vi "OperatorControlBox_XControl_Facade.vi"(0 "Data In":T4, 2 "Display State In":T2, 3 "Container State":T3) -> (6 "Data Out":T4, 7 "Display State Out":T2, 8 "Action":T1)   [LabVIEW 2018, in "OperatorControlBox_XControl.xctl"]
uses:
  OperatorControlBox_XControl.xctl
  OperatorControlBox_XControl_Data.ctl
  General/OperatorControlBox/TypeDefs/OperatorControlBoxButtons_Type.ctl
  <vilib>/_xctls/Container State.ctl
  OperatorControlBox_XControl_State.ctl
  <vilib>/_xctls/Action.ctl
  General/OperatorControlBox/TypeDefs/OperatorControlBoxButtonPosition_Type.ctl
  <vilib>/_xctls/XControlSupport.lvlib
panel:
  out "LED_Left":bool
  out "LED_Right":bool
  in  "Left_Right":bool
  out "LED_Cargo":bool
  out "LED_Hatch":bool
  in  "Hatch_Cargo":bool
  out "LED_Button4":bool
  in  "Button4":bool
  out "LED_Button3":bool
  in  "Button3":bool
  out "LED_Button2":bool
  in  "Button2":bool
  out "LED_Button1":bool
  in  "Button1":bool
  out "LED_Switch1_Right":bool
  out "LED_Switch1_Left":bool
  in  "Switch1":bool
  out "LED_Switch2_Right":bool
  out "LED_Switch2_Left":bool
  in  "Switch2":bool
  out "LED_Climb":bool
  in  "Climb":bool
  out "LED_CargoShip":bool
  in  "CargoShip":bool
  out "LED_Depot":bool
  in  "Depot":bool
  out "LED_FeederStation":bool
  in  "FeederStation":bool
  out "LED_NearRocketHigh":bool
  in  "NearRocketHigh":bool
  out "LED_NearRocketMid":bool
  in  "NearRocketMid":bool
  out "LED_NearRocketLow":bool
  in  "NearRocketLow":bool
  out "LED_FarRocketHigh":bool
  in  "FarRocketHigh":bool
  out "LED_FarRocketMid":bool
  in  "FarRocketMid":bool
  out "LED_FarRocketLow":bool
  in  "FarRocketLow":bool
  # "Left"
  # "Right"
  # "Hatch"
  # "Cargo"
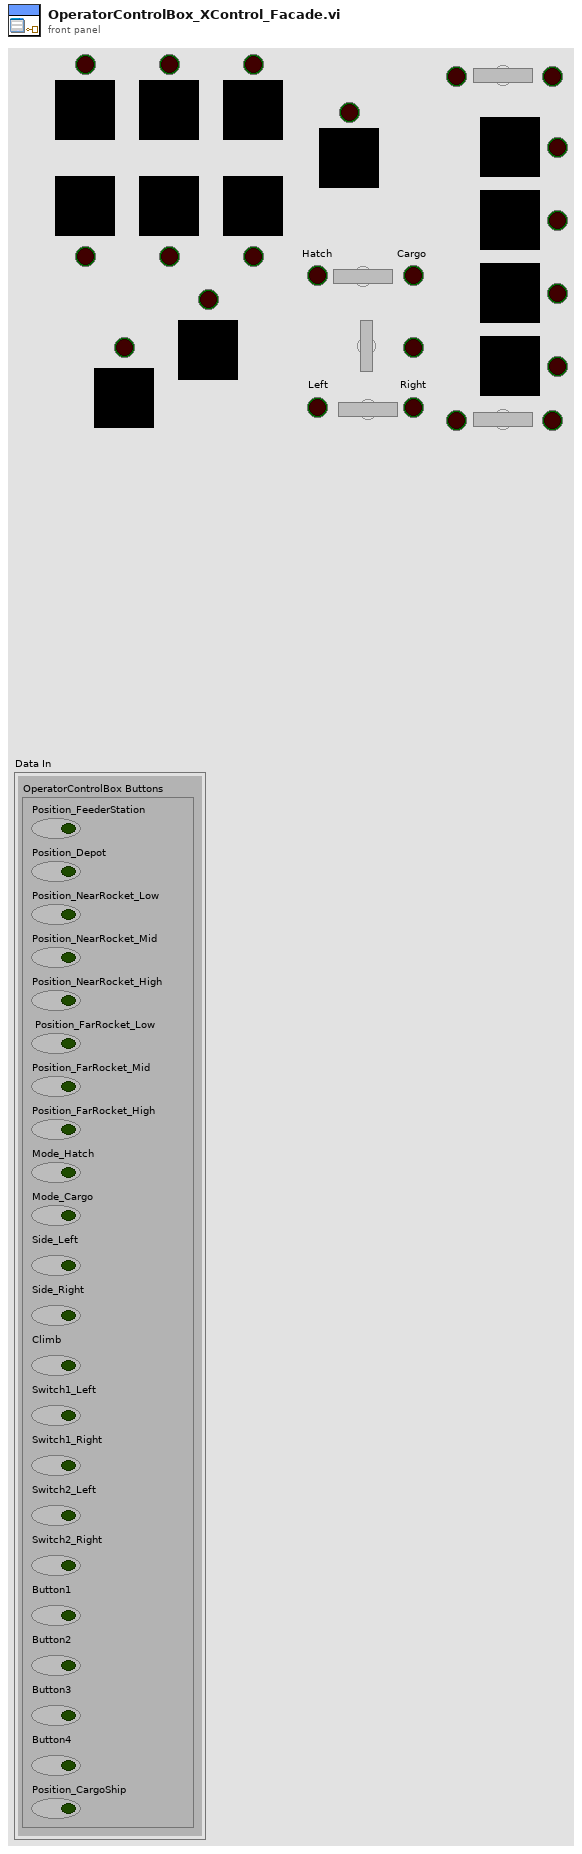
[diagram p1: front panel]
types:
  T1 = typedef "XControlSupport.lvlib/Action.ctl" = cluster{"Data Changed?":bool, "State Changed?":bool, "Action Name":string}
  T2 = typedef "OperatorControlBox_XControl.xctl/OperatorControlBox_XControl_State.ctl" = cluster{"Numeric":dbl}
  T3 = typedef "XControlSupport.lvlib/Container State.ctl" = cluster{"Indicator?":bool, "Run Mode?":bool, " Refnum":refnum<vi>}
  T4 = typedef "OperatorControlBox_XControl.xctl/OperatorControlBox_XControl_Data.ctl" = cluster{"OperatorControlBox Buttons":T5}
  T5 = typedef "OperatorControlBoxButtons_Type.ctl" = cluster{"Position_FeederStation":bool, "Position_Depot":bool, "Position_NearRocket_Low":bool, "Position_NearRocket_Mid":bool, "Position_NearRocket_High":bool, " Position_FarRocket_Low":bool, "Position_FarRocket_Mid":bool, "Position_FarRocket_High":bool, "Mode_Hatch":bool, "Mode_Cargo":bool, "Side_Left":bool, "Side_Right":bool, "Climb":bool, "Switch1_Left":bool, "Switch1_Right":bool, "Switch2_Left":bool, "Switch2_Right":bool, "Button1":bool, "Button2":bool, "Button3":bool, "Button4":bool, "Position_CargoShip":bool}
  T6 = typedef "OperatorControlBoxButtonPosition_Type.ctl" = enum16{"Unknown", "FeederStation", "Depot", "NearRocketLow", "NearRocketMid", "NearRocketHigh", "FarRocketLow", "FarRocketMid", "FarRocketHigh", "CargoShip"}
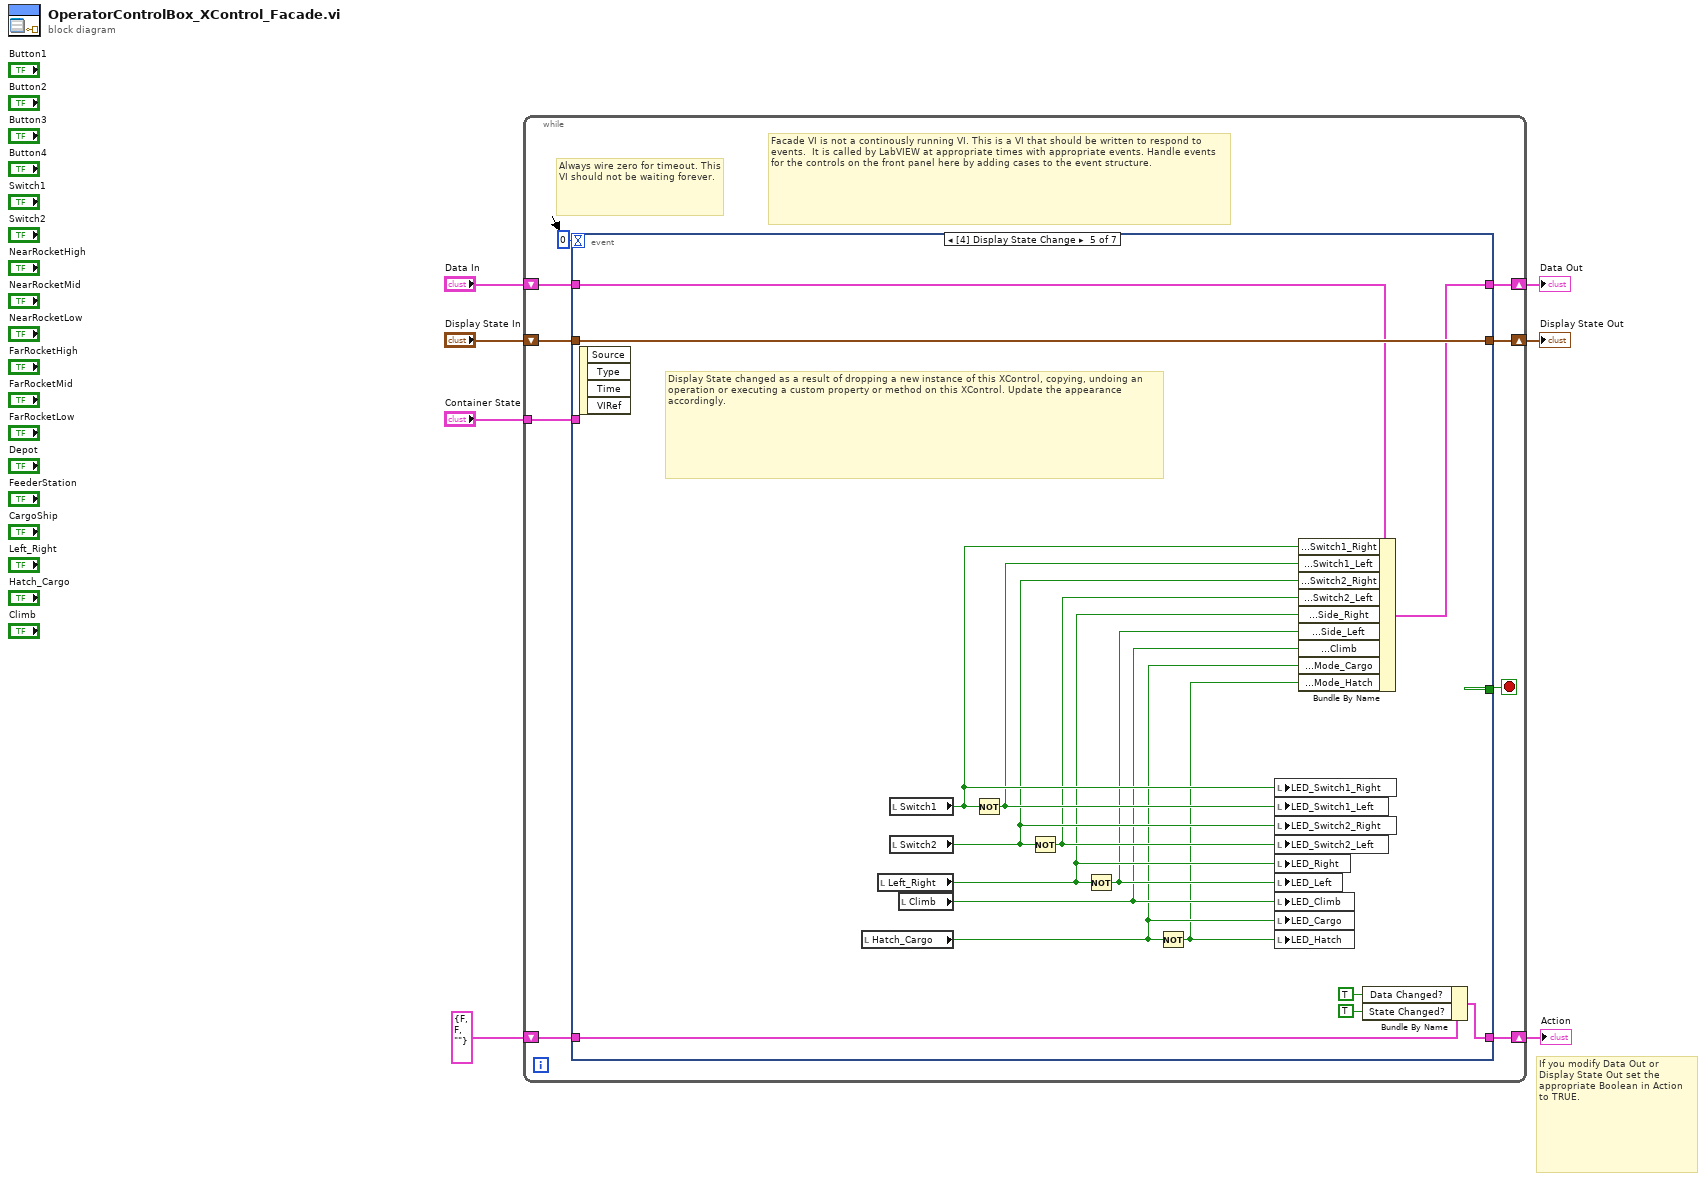
[diagram p0: block diagram]
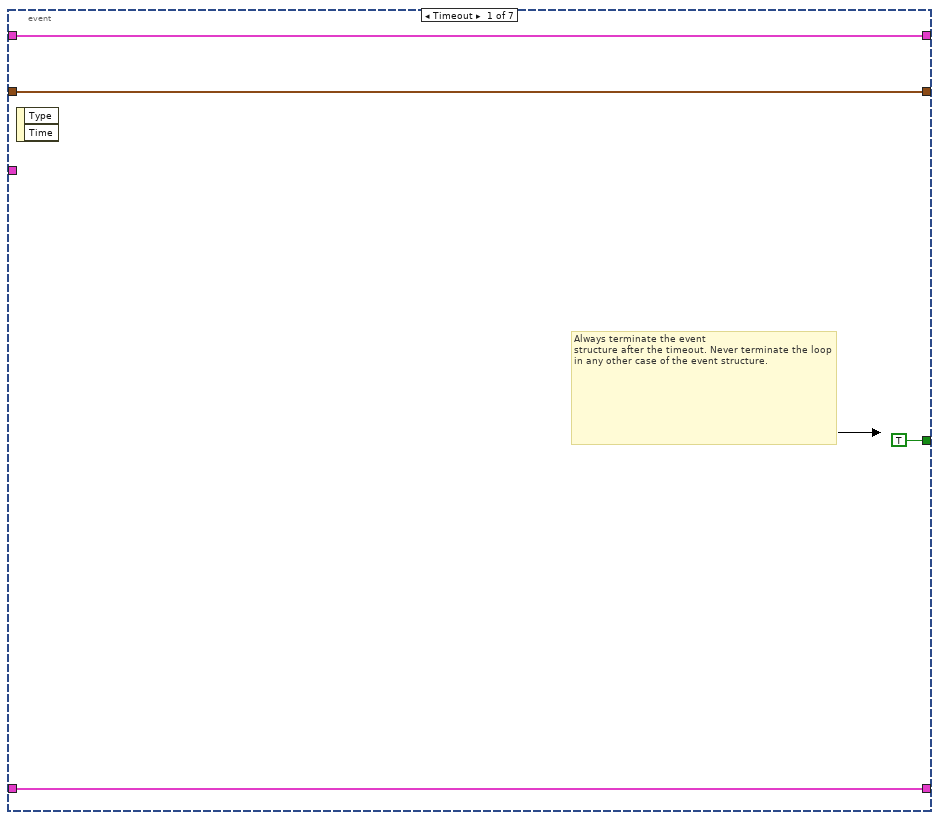
[diagram p2: hidden frame]
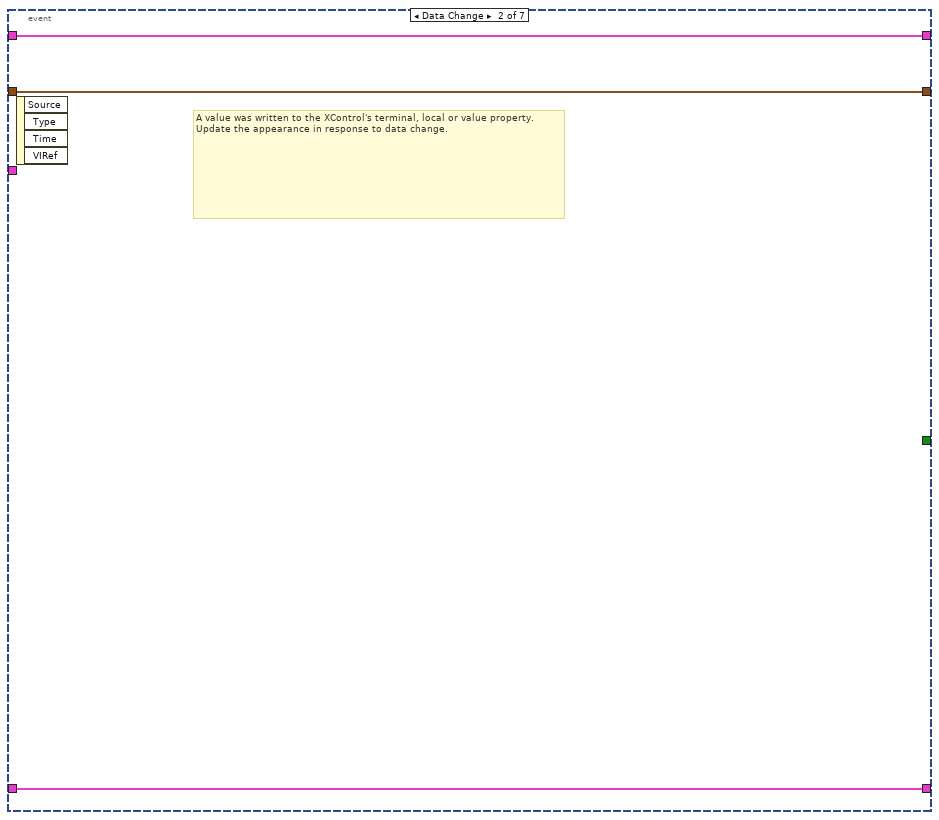
[diagram p3: hidden frame]
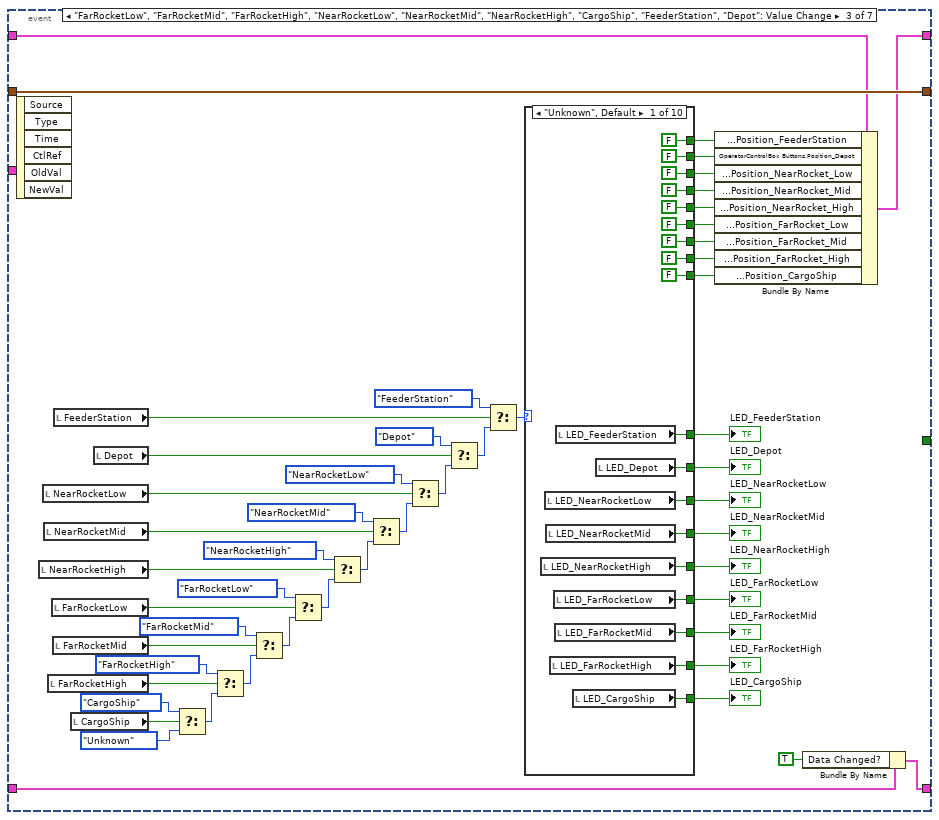
[diagram p4: hidden frame]
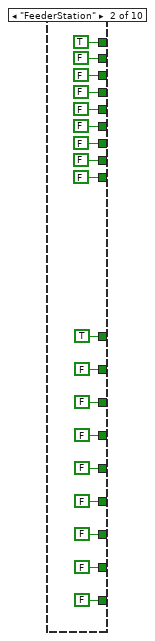
[diagram p5: hidden frame]
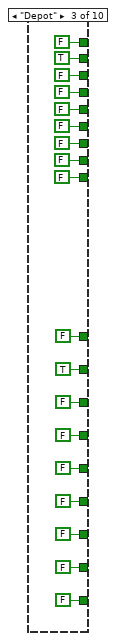
[diagram p6: hidden frame]
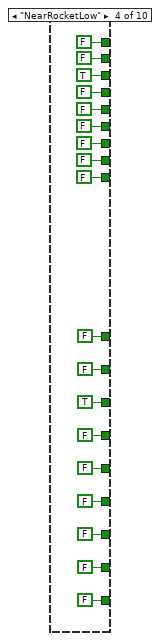
[diagram p7: hidden frame]
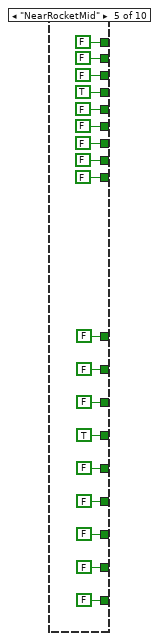
[diagram p8: hidden frame]
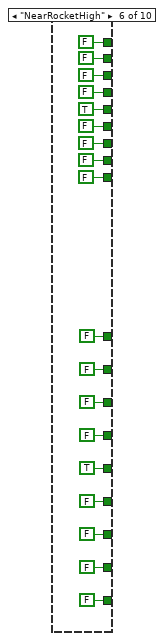
[diagram p9: hidden frame]
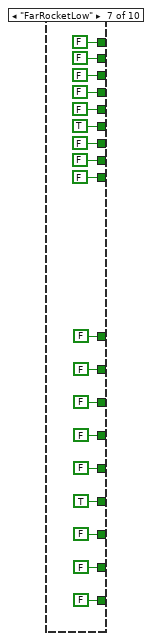
[diagram p10: hidden frame]
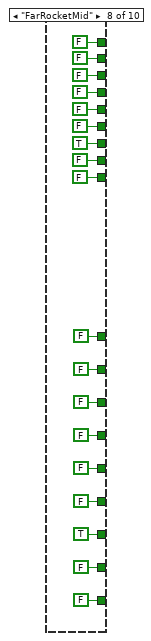
[diagram p11: hidden frame]
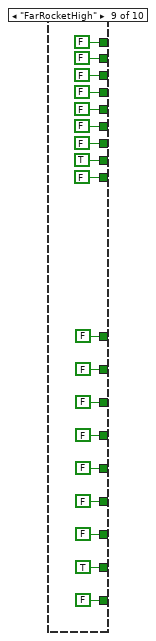
[diagram p12: hidden frame]
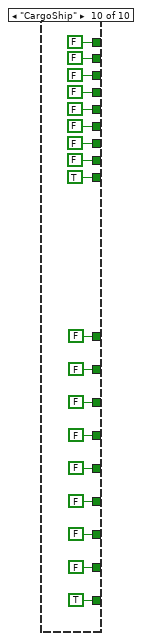
[diagram p13: hidden frame]
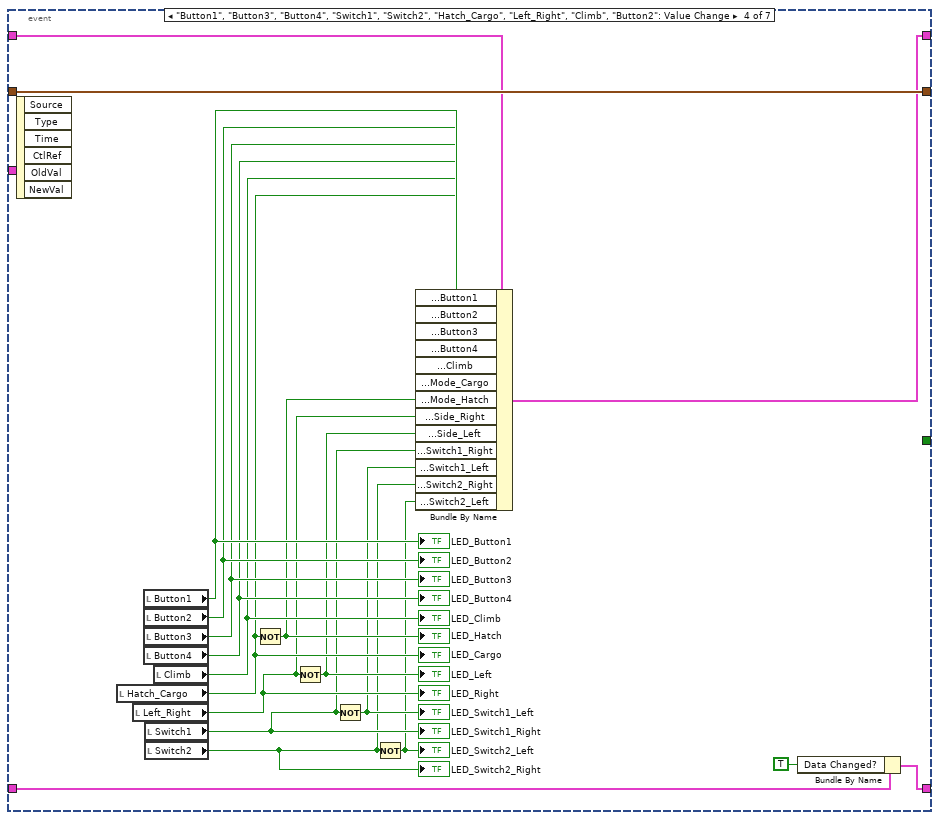
[diagram p14: hidden frame]
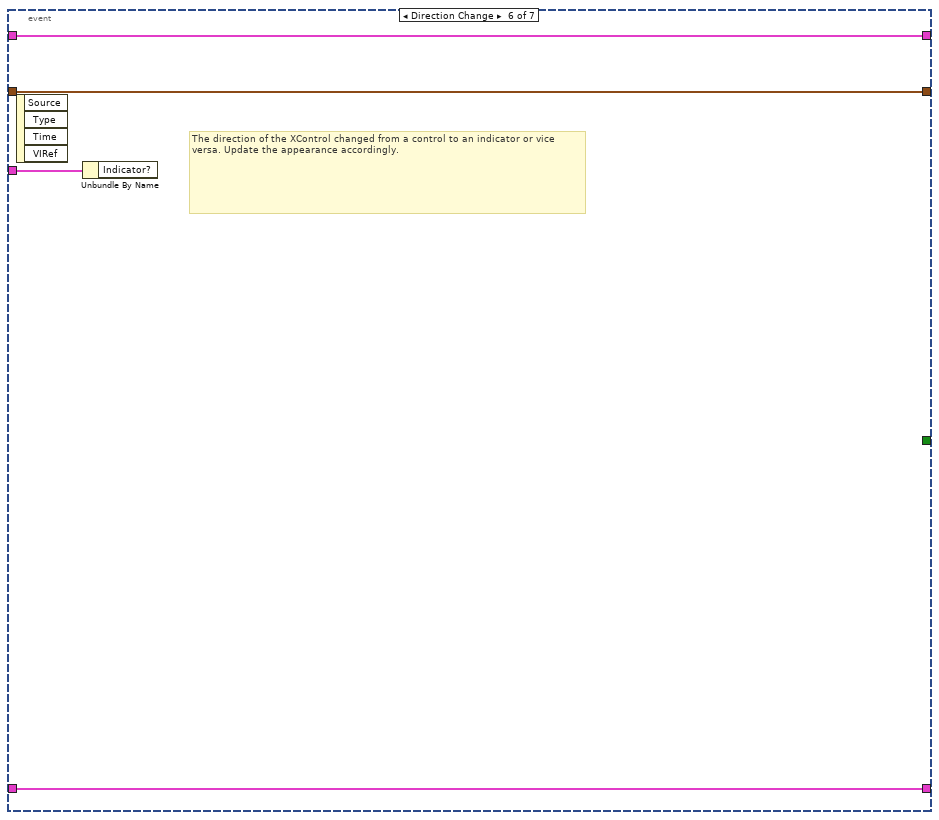
[diagram p15: hidden frame]
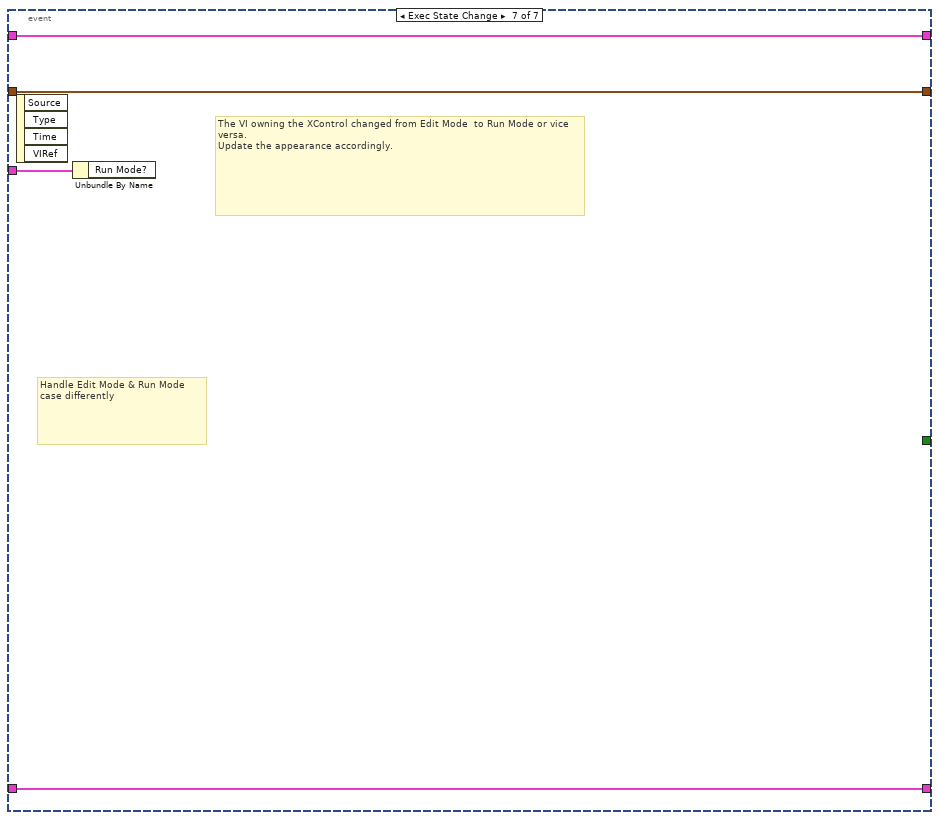
[diagram p16: hidden frame]
diagram:
  # "If you modify Data Out or\nDisplay State Out set the\nappropriate Boolean in Action\nto TRUE."
  n1 = while {
    shift-right: [w15] -> w4
    shift-left: "Display State In" -> [w16]
    tunnel: "Container State" -> [w12]
    shift-right: [w10] -> w7
    shift-left: "Data In" -> [w11]
    shift-right: [w8] -> w2
    shift-left: T1 {"Data Changed?"=FALSE, "State Changed?"=FALSE, "Action Name"=""} ("Action") -> [w9]
    stop <- w14 stop-if-true
    # "Facade VI is not a continously running VI. This is a VI that should be written to respond to events.  It is called by LabVIEW at appropriate times with appropriate events. Handle events for the controls on the front panel here by adding cases to the event structure."
    # "Always wire zero for timeout. This\nVI should not be waiting forever."
    n2 = event shown="[4] Display State Change" {
      selector: _ -> [_ _ _ _ _ _ _]
      dyn-events: _ -> [_ _ _ _ _ _ _]
      timeout: 0 -> [_ _ _ _ _ _ _]
      tunnel: w16 -> [w18 w22 w75 w274 w290 w293 w297]
      tunnel: [w18 w22 w75 w274 w290 w293 w297] -> w15
      tunnel: [TRUE _ _ _ _ _ _] -> w14
      tunnel: w12 -> [_ _ _ _ _ w294 w298]
      tunnel: w11 -> [w17 w23 w50 w273 w289 w292 w296]
      tunnel: [w17 w23 w49 w272 w288 w292 w296] -> w10
      tunnel: [w19 w21 w25 w256 w275 w291 w295] -> w8
      tunnel: w9 -> [w19 w21 w26 w257 w276 w291 w295]
      event Timeout {
        # "Always terminate the event\nstructure after the timeout. Never terminate the loop in any other case of the event structure."
        n3 = event-data() -> ()  [unwired: 1 in, 2 out]
      }
      event Data Change {
        # "A value was written to the XControl's terminal, local or value property.\nUpdate the appearance in response to data change."
        n4 = event-data() -> ()  [unwired: 1 in, 4 out]
      }
      event "FarRocketLow", "FarRocketMid", "FarRocketHigh", "NearRocketLow", "NearRocketMid", "NearRocketHigh", "CargoShip", "FeederStation", "Depot": Value Change {
        n5 = event-data() -> ()  [unwired: 1 in, 6 out]
        n6 = local read "NearRocketHigh"() -> (w56:bool)
        n7 = local read "NearRocketLow"() -> (w54:bool)
        n8 = local read "NearRocketMid"() -> (w55:bool)
        n9 = local read "FarRocketHigh"() -> (w74:bool)
        n10 = local read "FarRocketLow"() -> (w57:bool)
        n11 = local read "FarRocketMid"() -> (w58:bool)
        n12 = local read "FeederStation"() -> (w52:bool)
        n13 = local read "CargoShip"() -> (w30:bool)
        n14 = local read "Depot"() -> (w53:bool)
        n15 = Select(t=OperatorControlBoxButtonPosition_Type."CargoShip", s=w30, f=OperatorControlBoxButtonPosition_Type."Unknown") -> (s? t:f=w28:T6)
        n16 = Select(t=OperatorControlBoxButtonPosition_Type."FarRocketHigh", s=w74, f=w28) -> (s? t:f=w71:T6)
        n17 = Select(t=OperatorControlBoxButtonPosition_Type."FarRocketMid", s=w58, f=w71) -> (s? t:f=w69:T6)
        n18 = Select(t=OperatorControlBoxButtonPosition_Type."FarRocketLow", s=w57, f=w69) -> (s? t:f=w67:T6)
        n19 = Select(t=OperatorControlBoxButtonPosition_Type."NearRocketHigh", s=w56, f=w67) -> (s? t:f=w65:T6)
        n20 = Select(t=OperatorControlBoxButtonPosition_Type."NearRocketMid", s=w55, f=w65) -> (s? t:f=w63:T6)
        n21 = Select(t=OperatorControlBoxButtonPosition_Type."NearRocketLow", s=w54, f=w63) -> (s? t:f=w61:T6)
        n22 = Select(t=OperatorControlBoxButtonPosition_Type."Depot", s=w53, f=w61) -> (s? t:f=w59:T6)
        n23 = Select(t=OperatorControlBoxButtonPosition_Type."FeederStation", s=w52, f=w59) -> (s? t:f=w51:T6)
        n24 = case shown="\"Unknown\", Default" w51 {
          tunnel: [FALSE ("OperatorControlBox Buttons.Position_FeederStation") TRUE ("OperatorControlBox Buttons.Position_FeederStation") FALSE ("OperatorControlBox Buttons.Position_FeederStation") FALSE ("OperatorControlBox Buttons.Position_FeederStation") FALSE ("OperatorControlBox Buttons.Position_FeederStation") FALSE ("OperatorControlBox Buttons.Position_FeederStation") FALSE ("OperatorControlBox Buttons.Position_FeederStation") FALSE ("OperatorControlBox Buttons.Position_FeederStation") FALSE ("OperatorControlBox Buttons.Position_FeederStation") FALSE ("OperatorControlBox Buttons.Position_FeederStation")] -> w48
          tunnel: [FALSE ("OperatorControlBox Buttons.Position_FeederStation") FALSE ("OperatorControlBox Buttons.Position_FeederStation") TRUE ("OperatorControlBox Buttons.Position_FeederStation") FALSE ("OperatorControlBox Buttons.Position_FeederStation") FALSE ("OperatorControlBox Buttons.Position_FeederStation") FALSE ("OperatorControlBox Buttons.Position_FeederStation") FALSE ("OperatorControlBox Buttons.Position_FeederStation") FALSE ("OperatorControlBox Buttons.Position_FeederStation") FALSE ("OperatorControlBox Buttons.Position_FeederStation") FALSE ("OperatorControlBox Buttons.Position_FeederStation")] -> w47
          tunnel: [FALSE ("OperatorControlBox Buttons.Position_FeederStation") FALSE ("OperatorControlBox Buttons.Position_FeederStation") FALSE ("OperatorControlBox Buttons.Position_FeederStation") TRUE ("OperatorControlBox Buttons.Position_FeederStation") FALSE ("OperatorControlBox Buttons.Position_FeederStation") FALSE ("OperatorControlBox Buttons.Position_FeederStation") FALSE ("OperatorControlBox Buttons.Position_FeederStation") FALSE ("OperatorControlBox Buttons.Position_FeederStation") FALSE ("OperatorControlBox Buttons.Position_FeederStation") FALSE ("OperatorControlBox Buttons.Position_FeederStation")] -> w46
          tunnel: [FALSE ("OperatorControlBox Buttons.Position_FeederStation") FALSE ("OperatorControlBox Buttons.Position_FeederStation") FALSE ("OperatorControlBox Buttons.Position_FeederStation") FALSE ("OperatorControlBox Buttons.Position_FeederStation") TRUE ("OperatorControlBox Buttons.Position_FeederStation") FALSE ("OperatorControlBox Buttons.Position_FeederStation") FALSE ("OperatorControlBox Buttons.Position_FeederStation") FALSE ("OperatorControlBox Buttons.Position_FeederStation") FALSE ("OperatorControlBox Buttons.Position_FeederStation") FALSE ("OperatorControlBox Buttons.Position_FeederStation")] -> w45
          tunnel: [FALSE ("OperatorControlBox Buttons.Position_FeederStation") FALSE ("OperatorControlBox Buttons.Position_FeederStation") FALSE ("OperatorControlBox Buttons.Position_FeederStation") FALSE ("OperatorControlBox Buttons.Position_FeederStation") FALSE ("OperatorControlBox Buttons.Position_FeederStation") TRUE ("OperatorControlBox Buttons.Position_FeederStation") FALSE ("OperatorControlBox Buttons.Position_FeederStation") FALSE ("OperatorControlBox Buttons.Position_FeederStation") FALSE ("OperatorControlBox Buttons.Position_FeederStation") FALSE ("OperatorControlBox Buttons.Position_FeederStation")] -> w44
          tunnel: [FALSE ("OperatorControlBox Buttons.Position_FeederStation") FALSE ("OperatorControlBox Buttons.Position_FeederStation") FALSE ("OperatorControlBox Buttons.Position_FeederStation") FALSE ("OperatorControlBox Buttons.Position_FeederStation") FALSE ("OperatorControlBox Buttons.Position_FeederStation") FALSE ("OperatorControlBox Buttons.Position_FeederStation") TRUE ("OperatorControlBox Buttons.Position_FeederStation") FALSE ("OperatorControlBox Buttons.Position_FeederStation") FALSE ("OperatorControlBox Buttons.Position_FeederStation") FALSE ("OperatorControlBox Buttons.Position_FeederStation")] -> w43
          tunnel: [FALSE ("OperatorControlBox Buttons.Position_FeederStation") FALSE ("OperatorControlBox Buttons.Position_FeederStation") FALSE ("OperatorControlBox Buttons.Position_FeederStation") FALSE ("OperatorControlBox Buttons.Position_FeederStation") FALSE ("OperatorControlBox Buttons.Position_FeederStation") FALSE ("OperatorControlBox Buttons.Position_FeederStation") FALSE ("OperatorControlBox Buttons.Position_FeederStation") TRUE ("OperatorControlBox Buttons.Position_FeederStation") FALSE ("OperatorControlBox Buttons.Position_FeederStation") FALSE ("OperatorControlBox Buttons.Position_FeederStation")] -> w42
          tunnel: [FALSE ("OperatorControlBox Buttons.Position_FeederStation") FALSE ("OperatorControlBox Buttons.Position_FeederStation") FALSE ("OperatorControlBox Buttons.Position_FeederStation") FALSE ("OperatorControlBox Buttons.Position_FeederStation") FALSE ("OperatorControlBox Buttons.Position_FeederStation") FALSE ("OperatorControlBox Buttons.Position_FeederStation") FALSE ("OperatorControlBox Buttons.Position_FeederStation") FALSE ("OperatorControlBox Buttons.Position_FeederStation") TRUE ("OperatorControlBox Buttons.Position_FeederStation") FALSE ("OperatorControlBox Buttons.Position_FeederStation")] -> w41
          tunnel: [FALSE ("OperatorControlBox Buttons.Position_FeederStation") FALSE ("OperatorControlBox Buttons.Position_FeederStation") FALSE ("OperatorControlBox Buttons.Position_FeederStation") FALSE ("OperatorControlBox Buttons.Position_FeederStation") FALSE ("OperatorControlBox Buttons.Position_FeederStation") FALSE ("OperatorControlBox Buttons.Position_FeederStation") FALSE ("OperatorControlBox Buttons.Position_FeederStation") FALSE ("OperatorControlBox Buttons.Position_FeederStation") FALSE ("OperatorControlBox Buttons.Position_FeederStation") TRUE ("OperatorControlBox Buttons.Position_FeederStation")] -> w40
          tunnel: [w84 TRUE ("LED_FeederStation") FALSE ("LED_FeederStation") FALSE ("LED_FeederStation") FALSE ("LED_FeederStation") FALSE ("LED_FeederStation") FALSE ("LED_FeederStation") FALSE ("LED_FeederStation") FALSE ("LED_FeederStation") FALSE ("LED_FeederStation")] -> w39
          tunnel: [w83 FALSE ("LED_Depot") TRUE ("LED_Depot") FALSE ("LED_Depot") FALSE ("LED_Depot") FALSE ("LED_Depot") FALSE ("LED_Depot") FALSE ("LED_Depot") FALSE ("LED_Depot") FALSE ("LED_Depot")] -> w38
          tunnel: [w82 FALSE ("LED_NearRocketLow") FALSE ("LED_NearRocketLow") TRUE ("LED_NearRocketLow") FALSE ("LED_NearRocketLow") FALSE ("LED_NearRocketLow") FALSE ("LED_NearRocketLow") FALSE ("LED_NearRocketLow") FALSE ("LED_NearRocketLow") FALSE ("LED_NearRocketLow")] -> w37
          tunnel: [w81 FALSE ("LED_NearRocketMid") FALSE ("LED_NearRocketMid") FALSE ("LED_NearRocketMid") TRUE ("LED_NearRocketMid") FALSE ("LED_NearRocketMid") FALSE ("LED_NearRocketMid") FALSE ("LED_NearRocketMid") FALSE ("LED_NearRocketMid") FALSE ("LED_NearRocketMid")] -> w36
          tunnel: [w80 FALSE ("LED_NearRocketHigh") FALSE ("LED_NearRocketHigh") FALSE ("LED_NearRocketHigh") FALSE ("LED_NearRocketHigh") TRUE ("LED_NearRocketHigh") FALSE ("LED_NearRocketHigh") FALSE ("LED_NearRocketHigh") FALSE ("LED_NearRocketHigh") FALSE ("LED_NearRocketHigh")] -> w35
          tunnel: [w79 FALSE ("LED_FarRocketLow") FALSE ("LED_FarRocketLow") FALSE ("LED_FarRocketLow") FALSE ("LED_FarRocketLow") FALSE ("LED_FarRocketLow") TRUE ("LED_FarRocketLow") FALSE ("LED_FarRocketLow") FALSE ("LED_FarRocketLow") FALSE ("LED_FarRocketLow")] -> w34
          tunnel: [w78 FALSE ("LED_FarRocketMid") FALSE ("LED_FarRocketMid") FALSE ("LED_FarRocketMid") FALSE ("LED_FarRocketMid") FALSE ("LED_FarRocketMid") FALSE ("LED_FarRocketMid") TRUE ("LED_FarRocketMid") FALSE ("LED_FarRocketMid") FALSE ("LED_FarRocketMid")] -> w33
          tunnel: [w77 FALSE ("LED_FarRocketHigh") FALSE ("LED_FarRocketHigh") FALSE ("LED_FarRocketHigh") FALSE ("LED_FarRocketHigh") FALSE ("LED_FarRocketHigh") FALSE ("LED_FarRocketHigh") FALSE ("LED_FarRocketHigh") TRUE ("LED_FarRocketHigh") FALSE ("LED_FarRocketHigh")] -> w32
          tunnel: [w76 FALSE ("LED_CargoShip") FALSE ("LED_CargoShip") FALSE ("LED_CargoShip") FALSE ("LED_CargoShip") FALSE ("LED_CargoShip") FALSE ("LED_CargoShip") FALSE ("LED_CargoShip") FALSE ("LED_CargoShip") TRUE ("LED_CargoShip")] -> w31
          frame "Unknown", Default {
            n25 = local read "LED_NearRocketHigh"() -> (w80:bool)
            n26 = local read "LED_NearRocketLow"() -> (w82:bool)
            n27 = local read "LED_NearRocketMid"() -> (w81:bool)
            n28 = local read "LED_FarRocketHigh"() -> (w77:bool)
            n29 = local read "LED_FarRocketLow"() -> (w79:bool)
            n30 = local read "LED_FarRocketMid"() -> (w78:bool)
            n31 = local read "LED_FeederStation"() -> (w84:bool)
            n32 = local read "LED_CargoShip"() -> (w76:bool)
            n33 = local read "LED_Depot"() -> (w83:bool)
          }
          frame "FeederStation" {
          }
          frame "Depot" {
          }
          frame "NearRocketLow" {
          }
          frame "NearRocketMid" {
          }
          frame "NearRocketHigh" {
          }
          frame "FarRocketLow" {
          }
          frame "FarRocketMid" {
          }
          frame "FarRocketHigh" {
          }
          frame "CargoShip" {
          }
        }
        "LED_FarRocketLow" <- w34
        "LED_FarRocketMid" <- w33
        "LED_FarRocketHigh" <- w32
        "LED_NearRocketLow" <- w37
        "LED_FeederStation" <- w39
        "LED_CargoShip" <- w31
        "LED_NearRocketMid" <- w36
        "LED_NearRocketHigh" <- w35
        "LED_Depot" <- w38
        n34 = Bundle By Name(cluster=w50, "OperatorControlBox Buttons.Position_FeederStation"=w48, "OperatorControlBox Buttons.Position_Depot"=w47, "OperatorControlBox Buttons.Position_NearRocket_Low"=w46, "OperatorControlBox Buttons.Position_NearRocket_Mid"=w45, "OperatorControlBox Buttons.Position_NearRocket_High"=w44, "OperatorControlBox Buttons.Position_FarRocket_Low"=w43, "OperatorControlBox Buttons.Position_FarRocket_Mid"=w42, "OperatorControlBox Buttons.Position_FarRocket_High"=w41, "OperatorControlBox Buttons.Position_CargoShip"=w40) -> (w49:T4)
        n35 = Bundle By Name(cluster=w26, "Data Changed?"=TRUE) -> (w25:T1)
      }
      event "Button1", "Button3", "Button4", "Switch1", "Switch2", "Hatch_Cargo", "Left_Right", "Climb", "Button2": Value Change {
        n36 = event-data() -> ()  [unwired: 1 in, 6 out]
        n37 = local read "Hatch_Cargo"() -> (w266:bool)
        "LED_Cargo" <- w266
        n38 = local read "Left_Right"() -> (w264:bool)
        "LED_Right" <- w264
        n39 = local read "Button1"() -> (w271:bool)
        "LED_Button1" <- w271
        n40 = local read "Button2"() -> (w270:bool)
        "LED_Button2" <- w270
        n41 = local read "Button3"() -> (w269:bool)
        "LED_Button3" <- w269
        n42 = local read "Button4"() -> (w268:bool)
        "LED_Button4" <- w268
        n43 = local read "Switch1"() -> (w262:bool)
        "LED_Switch1_Right" <- w262
        n44 = local read "Switch2"() -> (w260:bool)
        "LED_Switch2_Right" <- w260
        n45 = local read "Climb"() -> (w267:bool)
        "LED_Climb" <- w267
        n46 = Not(x=w266) -> (.not. x?=w265:bool)
        "LED_Hatch" <- w265
        n47 = Not(x=w264) -> (.not. x?=w263:bool)
        "LED_Left" <- w263
        n48 = Not(x=w262) -> (.not. x?=w261:bool)
        "LED_Switch1_Left" <- w261
        n49 = Not(x=w260) -> (.not. x?=w259:bool)
        "LED_Switch2_Left" <- w259
        n50 = Bundle By Name(cluster=w273, "OperatorControlBox Buttons.Button1"=w271, "OperatorControlBox Buttons.Button2"=w270, "OperatorControlBox Buttons.Button3"=w269, "OperatorControlBox Buttons.Button4"=w268, "OperatorControlBox Buttons.Climb"=w267, "OperatorControlBox Buttons.Mode_Cargo"=w266, "OperatorControlBox Buttons.Mode_Hatch"=w265, "OperatorControlBox Buttons.Side_Right"=w264, "OperatorControlBox Buttons.Side_Left"=w263, "OperatorControlBox Buttons.Switch1_Right"=w262, "OperatorControlBox Buttons.Switch1_Left"=w261, "OperatorControlBox Buttons.Switch2_Right"=w260, "OperatorControlBox Buttons.Switch2_Left"=w259) -> (w272:T4)
        n51 = Bundle By Name(cluster=w257, "Data Changed?"=TRUE) -> (w256:T1)
      }
      event Display State Change {
        # "Display State changed as a result of dropping a new instance of this XControl, copying, undoing an operation or executing a custom property or method on this XControl. Update the appearance accordingly."
        n52 = event-data() -> ()  [unwired: 1 in, 4 out]
        n53 = local read "Hatch_Cargo"() -> (w280:bool)
        n54 = local read "Left_Right"() -> (w283:bool)
        n55 = local read "Switch1"() -> (w287:bool)
        n56 = local read "Switch2"() -> (w285:bool)
        n57 = local read "Climb"() -> (w281:bool)
        n58 = Not(x=w287) -> (.not. x?=w286:bool)
        n59 = Not(x=w285) -> (.not. x?=w284:bool)
        n60 = Not(x=w283) -> (.not. x?=w282:bool)
        n61 = Not(x=w280) -> (.not. x?=w279:bool)
        n62 = local write "LED_Switch1_Right"(w287) -> ()
        n63 = local write "LED_Switch1_Left"(w286) -> ()
        n64 = local write "LED_Switch2_Right"(w285) -> ()
        n65 = local write "LED_Switch2_Left"(w284) -> ()
        n66 = local write "LED_Right"(w283) -> ()
        n67 = local write "LED_Left"(w282) -> ()
        n68 = local write "LED_Climb"(w281) -> ()
        n69 = local write "LED_Cargo"(w280) -> ()
        n70 = local write "LED_Hatch"(w279) -> ()
        n71 = Bundle By Name(cluster=w289, "OperatorControlBox Buttons.Switch1_Right"=w287, "OperatorControlBox Buttons.Switch1_Left"=w286, "OperatorControlBox Buttons.Switch2_Right"=w285, "OperatorControlBox Buttons.Switch2_Left"=w284, "OperatorControlBox Buttons.Side_Right"=w283, "OperatorControlBox Buttons.Side_Left"=w282, "OperatorControlBox Buttons.Climb"=w281, "OperatorControlBox Buttons.Mode_Cargo"=w280, "OperatorControlBox Buttons.Mode_Hatch"=w279) -> (w288:T4)
        n72 = Bundle By Name(cluster=w276, "Data Changed?"=TRUE, "State Changed?"=TRUE) -> (w275:T1)
      }
      event Direction Change {
        # "The direction of the XControl changed from a control to an indicator or vice versa. Update the appearance accordingly."
        n73 = event-data() -> ()  [unwired: 1 in, 4 out]
        n74 = Unbundle By Name(w294) -> ()  [unwired: 1 out]
      }
      event Exec State Change {
        # "The VI owning the XControl changed from Edit Mode  to Run Mode or vice versa.\nUpdate the appearance accordingly."
        # "Handle Edit Mode & Run Mode\ncase differently"
        n75 = event-data() -> ()  [unwired: 1 in, 4 out]
        n76 = Unbundle By Name(w298) -> ()  [unwired: 1 out]
      }
    }
  }
  "Display State Out" <- w4
  "Data Out" <- w7
  "Action" <- w2
